vi "CT_SaveWaveformWithNames.vi"(1 "error in (no error)":errorcluster, 2 "delimiter (Tab)":string="\t", 3 "waveforms":waveform(dbl)[](array[waveform]), 4 "file path (dialog if empty)":path) -> (0 "error out":errorcluster)   [LabVIEW 2020]
panel:
  out "spreadsheet string":string
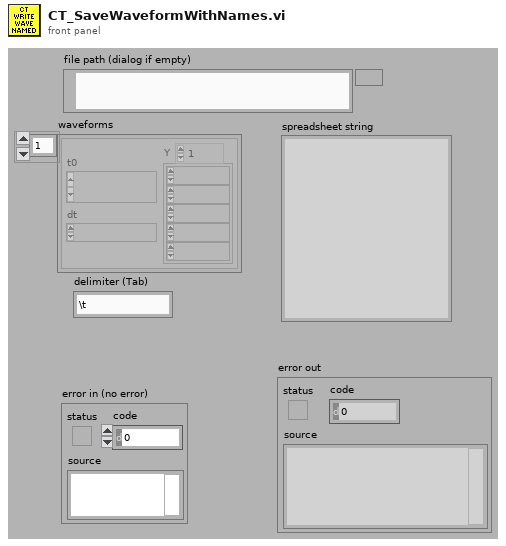
[diagram p1: front panel]
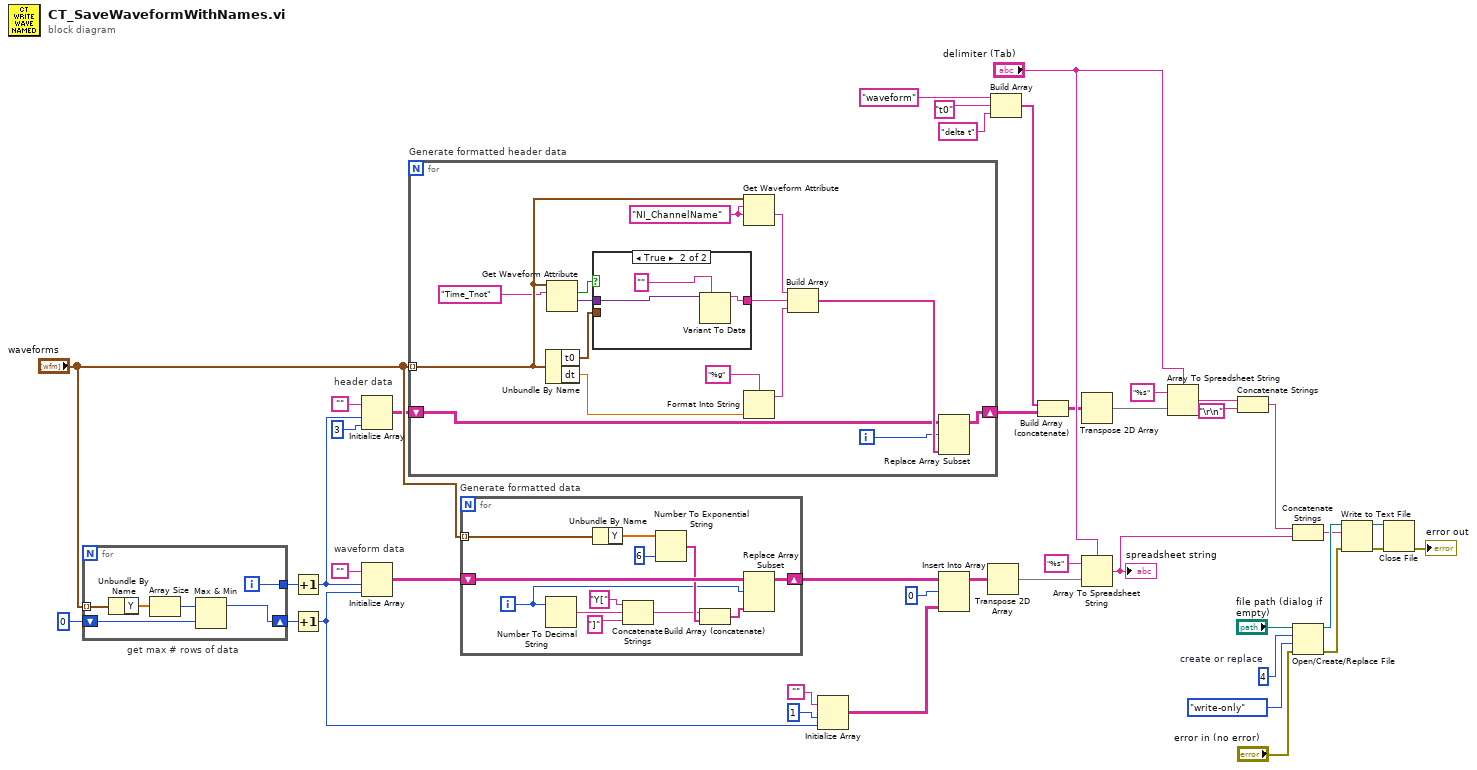
[diagram p0: block diagram]
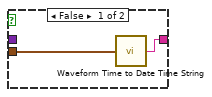
[diagram p2: hidden frame]
diagram:
  w9 = i16 4  # create or replace
  # "header data"
  # "waveform data"
  # "get max # rows of data"
  n1 = for {
    tunnel: "waveforms" -> [w48] mode=indexing
    shift-right: [w44] -> w36
    shift-left: 0 -> [w45]
    tunnel: [w43] -> w34
    i -> [w43]
    n2 = Unbundle By Name(w48) -> ("Y"=w47:dbl[])
    n3 = Array Size(array=w47) -> (size(s)=w46:i32)
    n4 = Max & Min(x=w46, y=w45) -> (max(x,y)=w44:i32)  [unwired: 1 out]
  }
  n5 = Increment(x=w34) -> (x+1=w33:i32)
  n6 = Increment(x=w36) -> (x+1=w16:i32)
  n7 = Initialize Array("", w33, 3 ("dimension size")) -> (w18:string[][])
  n8 = Initialize Array("", w33, w16) -> (w35:string[][])
  n9 = for "Generate formatted header data" {
    tunnel: "waveforms" -> [w54] mode=indexing
    shift-right: [w58] -> w23
    shift-left: w18 -> [w59]
    i -> [w57]
    w56 = "NI_ChannelName" ("name")
    n10 = Unbundle By Name(w54) -> ("t0"=w51:timestamp, "dt"=w62:dbl)
    n11 = Get Waveform Attribute(6:"Time_Tnot" ("name"), 7:w54) -> (1:w49:variant, 2:w52:bool)  [unwired: 2 in, 2 out]
    n12 = case shown="True" w52 {
      tunnel: w51 -> [w65 _]
      tunnel: [w64 w68] -> w50
      tunnel: w49 -> [_ w66]
      frame False {
        n13 = call <vilib>:"Waveform Time to Date Time String.vi"("t0"=w65) -> ("String"=w64:string)
      }
      frame True {
        n14 = Variant To Data(type="" ("name"), Variant=w66) -> (data=w68:string)  [unwired: 1 in, 1 out]
      }
    }
    n15 = Get Waveform Attribute(5:w56, 6:w56, 7:w54) -> (1:w55:string)  [unwired: 1 in, 3 out]
    n16 = Format Into String(format string="%g" ("Format String"), w62) -> (resulting string=w63:string)  [unwired: 2 in, 1 out]
    n17 = Build Array(w55, w50, w63) -> (w60:string[])
    n18 = Replace Array Subset(array=w59, new element=w60, index (row)=w57) -> (w58:string[][])  [unwired: 1 in]
  }
  n19 = for "Generate formatted data" {
    tunnel: "waveforms" -> [w78] mode=indexing
    shift-right: [w76] -> w13
    shift-left: w35 -> [w77]
    i -> [w69]
    n20 = Number To Decimal String(number=w69) -> (decimal integer string=w73:string)  [unwired: 1 in]
    n21 = Unbundle By Name(w78) -> ("Y"=w80:dbl[])
    n22 = Concatenate Strings("Y[", w73, "]") -> (w70:string)
    n23 = Number To Exponential String(number=w80, precision (6)=i16 6) -> (E-format string=w75:string[])  [unwired: 2 in]
    n24 = Build Array (concatenate)(w70, w75) -> (w74:string[])
    n25 = Replace Array Subset(array=w77, new element=w74, index (row)=w69) -> (w76:string[][])  [unwired: 1 in]
  }
  n26 = Initialize Array("", 1 ("dimension size"), w16) -> (w14:string[][])
  n27 = Insert Into Array(array=w13, index (row)=0, new element=w14) -> (w12:string[][])  [unwired: 1 in]
  n28 = Transpose 2D Array(2D array=w12) -> (transposed array=w31:string[][])
  n29 = Build Array("waveform", "t0", "delta t") -> (w24:string[])
  n30 = Build Array (concatenate)(w24, w23) -> (w21:string[][])
  n31 = Transpose 2D Array(2D array=w21) -> (transposed array=w22:string[][])
  n32 = Array To Spreadsheet String(delimiter (Tab)="delimiter (Tab)", array=w31, 3:"%s" ("format (%.3f)")) -> (spreadsheet string=w40:string)
  "spreadsheet string" <- w40
  n33 = Array To Spreadsheet String(delimiter (Tab)="delimiter (Tab)", array=w22, 3:"%s" ("format string")) -> (spreadsheet string=w26:string)
  n34 = Concatenate Strings(w26, "\r\n") -> (w39:string)
  n35 = Concatenate Strings(w39, w40) -> (w1:string)
  n36 = Open/Create/Replace File(file path (use dialog)="file path (dialog if empty)", error in="error in (no error)", operation (0:open)=w9, access (0:read/write)=enum16{"read/write", "read-only", "write-only"}."write-only") -> (refnum out=w5:refnum<file>, error out=w4:errorcluster)  [unwired: 2 in, 1 out]
  n37 = Write to Text File(file (use dialog)=w5, text=w1, error in=w4) -> (refnum out=w3:refnum<file>, error out=w2:errorcluster)  [unwired: 1 in, 1 out]
  n38 = Close File(refnum=w3, error in=w2) -> (error out=→"error out":errorcluster)  [unwired: 1 out]
